vi "configure dialog.vi"(9 "Channel":u32, 11 "Attributes in":T1[](array[typedef])) -> (1 "Channel out":u32, 2 "Cancelled?":bool, 3 "Attributes out":T1[](array[typedef]))   [LabVIEW 2020, in "Set DDT Attributes.lvlib"]
doc: "Sets the attributes of the dynamic data you wire to <B>Signals In</B>."
uses:
  <vilib>/express/express signal manip/GetorSetDDTAttributes/Set DDT Attributes/Set DDT Attributes.lvlib
  <vilib>/express/express signal manip/GetorSetDDTAttributes/Shared VIs/Attributes data.ctl
  <vilib>/express/express signal manip/GetorSetDDTAttributes/Shared VIs/Input.ctl
  <vilib>/express/express signal manip/GetorSetDDTAttributes/Shared VIs/Attributes name.ctl
  <vilib>/express/express signal manip/GetorSetDDTAttributes/Shared VIs/TimeType.ctl
  <vilib>/express/express signal manip/GetorSetDDTAttributes/Shared VIs/XDimension.ctl
  <vilib>/express/express signal manip/GetorSetDDTAttributes/Shared VIs/GetSetShared.lvlib
  <vilib>/express/express signal manip/GetorSetDDTAttributes/Set DDT Attributes/Set DDT Properties.xnode
panel:
  in  "Signal Index":u32
  in  "Start timestamp":bool
  in  "Unit":bool
  in  "X dimension":bool
  in  "Timestamp":bool
  in  "Time mode":bool
  in  "Signal name":bool
  in  "Timestamp value":timestamp
  in  "Start timestamp value":timestamp
  in  "Unit value":string
  in  "Time mode value":u16(ring)=1 items=["Absolute", "Relative"]
  in  "X dimension value":u16(ring)=1 items=["No Unit [-]", "Time [sec]", "Frequency [Hz]"]
  in  "Signal name value":string
  in  "help":bool
  in  "Cancel":bool
  in  "OK":bool
  # "All Signals"
  # "Value"
  # "Value"
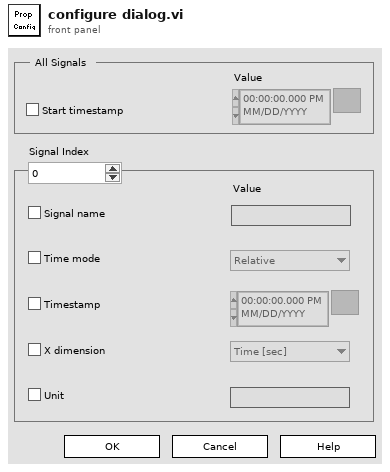
[diagram p1: front panel]
types:
  T1 = typedef "GetSetShared.lvlib/Attributes data.ctl" = cluster{"State":T2, "Attributes Name":T3, "Value":variant, "wired?":bool}
  T2 = typedef "GetSetShared.lvlib/Input.ctl" = bool
  T3 = typedef "GetSetShared.lvlib/Attributes name.ctl" = enum16{"NI_ChannelName", "NI_ExpIsRelativeTime", "NI_ExpTimeStamp", "NI_ExpStartTimeStamp", "NI_ExpXDimension", "NI_UnitDescription"}
  T4 = typedef "GetSetShared.lvlib/TimeType.ctl" = enum16{"Absolute", "Relative"}
  T5 = typedef "GetSetShared.lvlib/XDimension.ctl" = enum16{"No Unit [-]", "Time [sec]", "Frequency [Hz]"}
  T6 = cluster{"Description":string, "Path":path, "Tag":string}
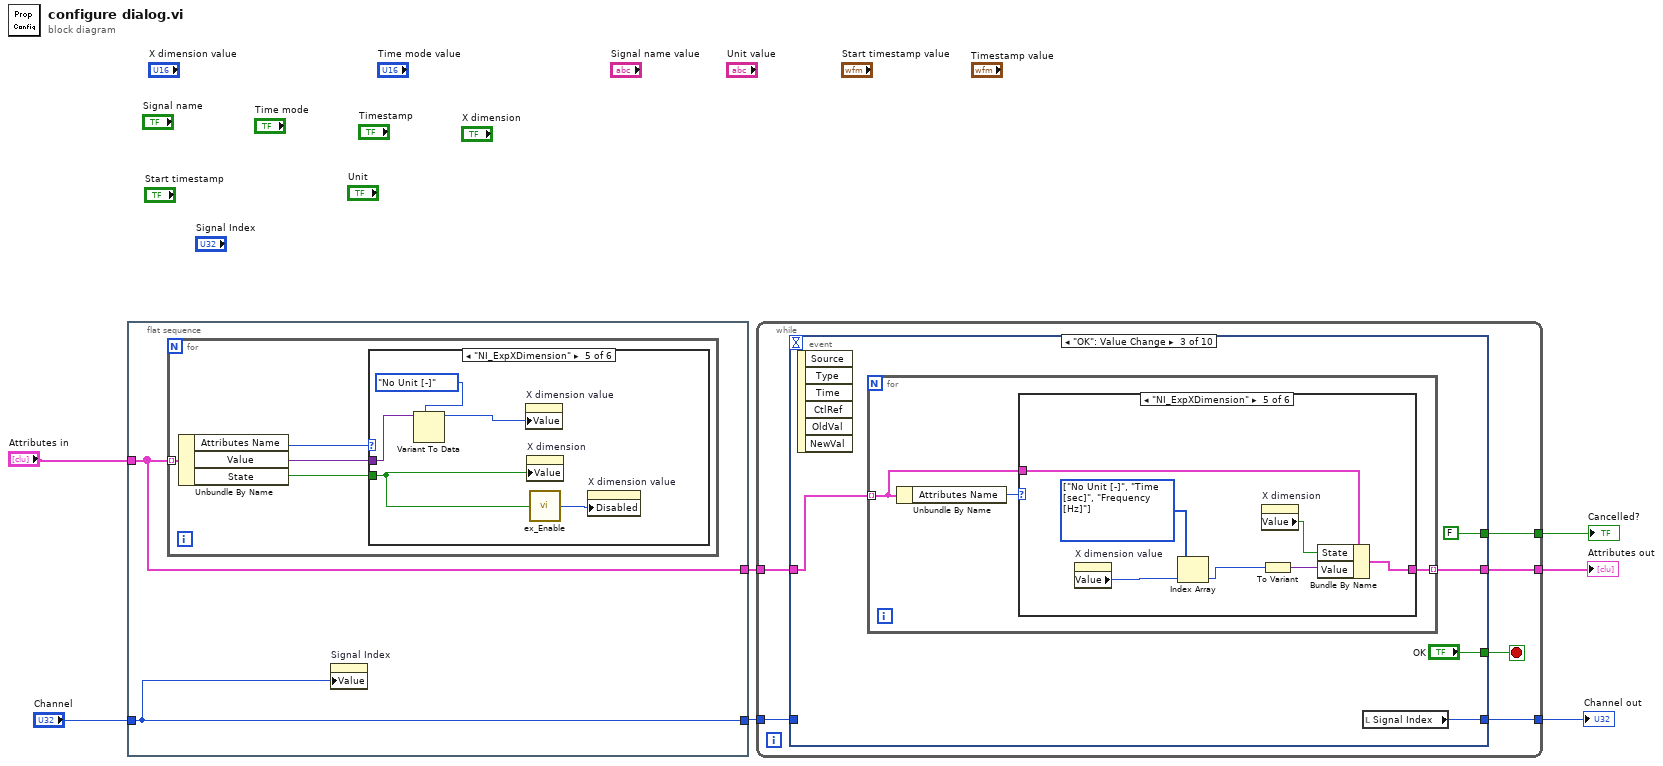
[diagram p0: block diagram]
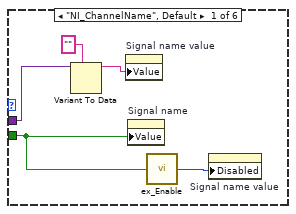
[diagram p2: hidden frame]
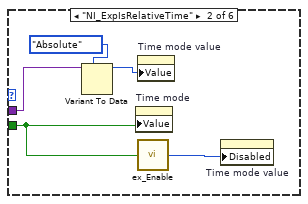
[diagram p3: hidden frame]
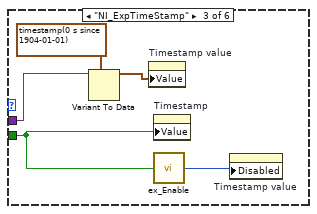
[diagram p4: hidden frame]
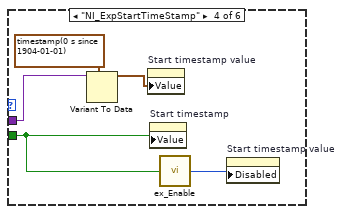
[diagram p5: hidden frame]
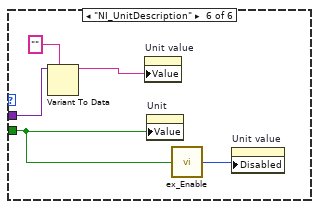
[diagram p6: hidden frame]
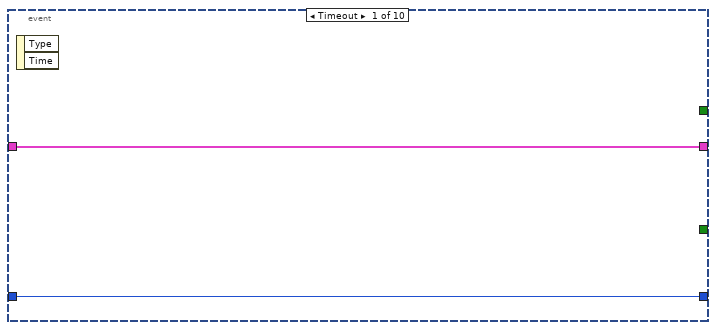
[diagram p7: hidden frame]
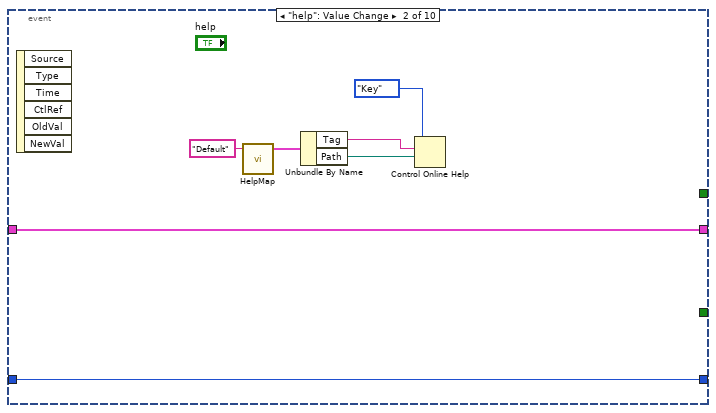
[diagram p8: hidden frame]
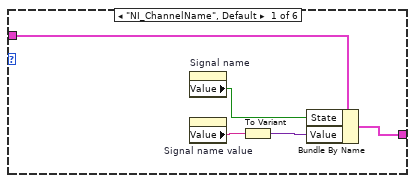
[diagram p9: hidden frame]
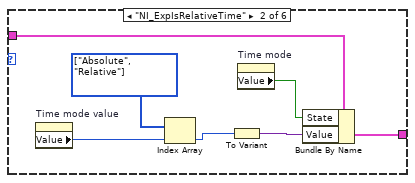
[diagram p10: hidden frame]
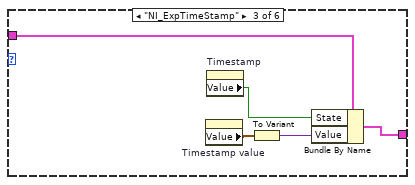
[diagram p11: hidden frame]
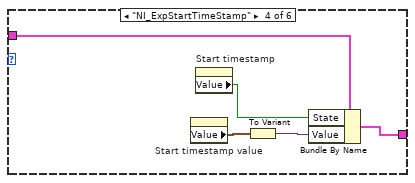
[diagram p12: hidden frame]
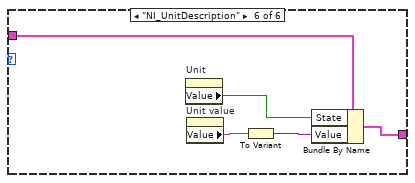
[diagram p13: hidden frame]
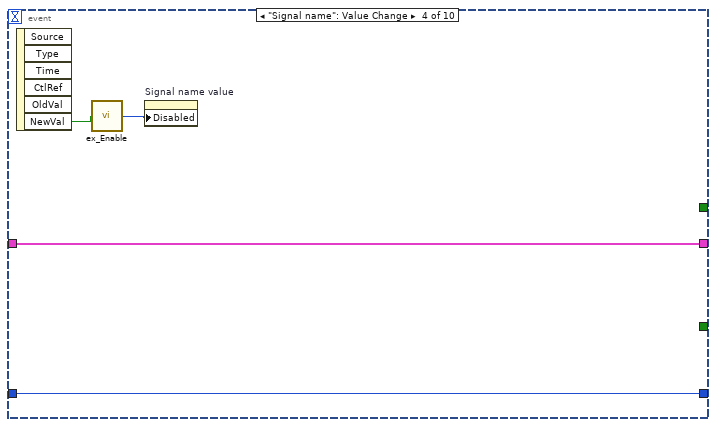
[diagram p14: hidden frame]
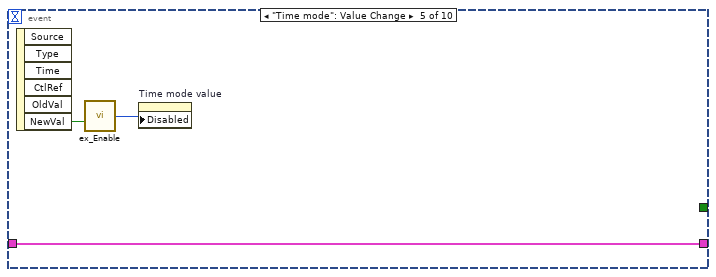
[diagram p15: hidden frame]
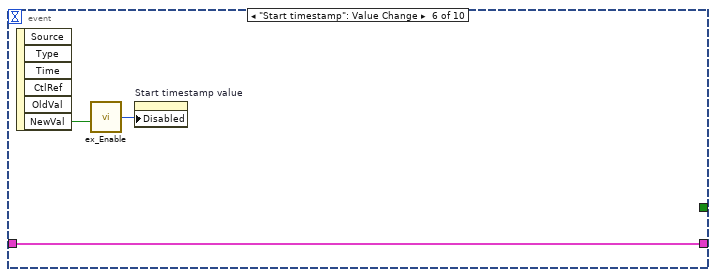
[diagram p16: hidden frame]
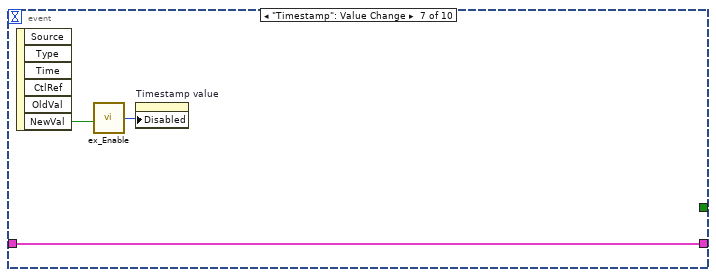
[diagram p17: hidden frame]
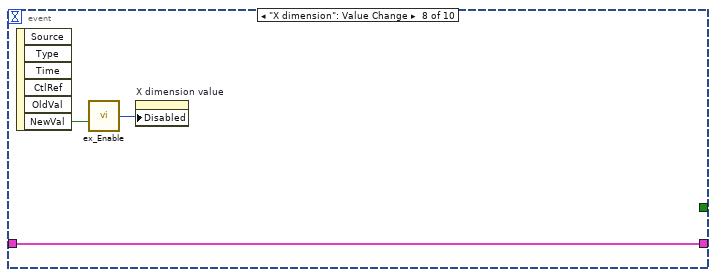
[diagram p18: hidden frame]
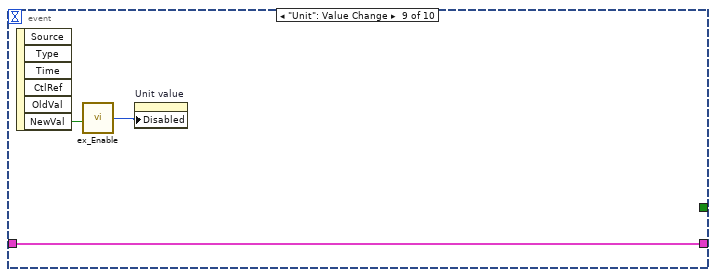
[diagram p19: hidden frame]
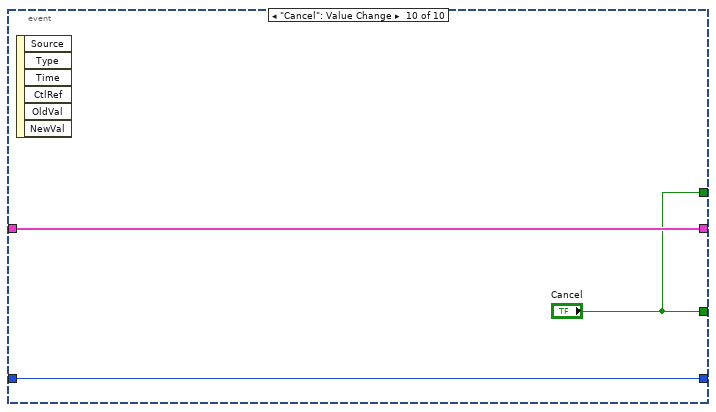
[diagram p20: hidden frame]
diagram:
  n1 = flat-sequence {
    tunnel: "Attributes in" -> [w9]
    tunnel: [w9] -> w4
    tunnel: "Channel" -> [w8]
    tunnel: [w8] -> w3
    frame #0 {
      n2 = for {
        tunnel: w9 -> [w13] mode=indexing
        n3 = Unbundle By Name(w13) -> ("Attributes Name"=w12:T3, "Value"=w11:variant, "State"=w10:T2)
        n4 = case shown="\"NI_ExpXDimension\"" w12 {
          tunnel: w11 -> [w18 w23 w28 w32 w38 w43]
          tunnel: w10 -> [w14 w21 w24 w29 w34 w39]
          frame "NI_ChannelName", Default {
            n5 = Variant To Data(type="", Variant=w18) -> (data=w16:string)  [unwired: 1 in, 1 out]
            n6 = property on="Signal name value" class="Str"("Value"=w16) -> ()  [unwired: 2 in, 2 out]
            n7 = property on="Signal name" class="Bool (strict)"("Value"=w14) -> ()  [unwired: 2 in, 2 out]
            n8 = call <vilib>:"ex_Enable.vi"("Enable?"=w14) -> ("Disabled Value"=w15:u8)
            n9 = property on="Signal name value" class="Str"("Disabled"=w15) -> ()  [unwired: 2 in, 2 out]
          }
          frame "NI_ExpIsRelativeTime" {
            n10 = Variant To Data(type=TimeType."Absolute" ("RelativeTime?"), Variant=w23) -> (data=w19:T4)  [unwired: 1 in, 1 out]
            n11 = property on="Time mode" class="Bool (strict)"("Value"=w21) -> ()  [unwired: 2 in, 2 out]
            n12 = property on="Time mode value" class="Ring (strict)"("Value"=w19) -> ()  [unwired: 2 in, 2 out]
            n13 = call <vilib>:"ex_Enable.vi"("Enable?"=w21) -> ("Disabled Value"=w22:u8)
            n14 = property on="Time mode value" class="Ring (strict)"("Disabled"=w22) -> ()  [unwired: 2 in, 2 out]
          }
          frame "NI_ExpTimeStamp" {
            n15 = Variant To Data(type=timestamp(0 s since 1904-01-01), Variant=w28) -> (data=w26:timestamp)  [unwired: 1 in, 1 out]
            n16 = property on="Timestamp value" class="AbsTime (strict)"("Value"=w26) -> ()  [unwired: 2 in, 2 out]
            n17 = property on="Timestamp" class="Bool (strict)"("Value"=w24) -> ()  [unwired: 2 in, 2 out]
            n18 = call <vilib>:"ex_Enable.vi"("Enable?"=w24) -> ("Disabled Value"=w25:u8)
            n19 = property on="Timestamp value" class="AbsTime (strict)"("Disabled"=w25) -> ()  [unwired: 2 in, 2 out]
          }
          frame "NI_ExpStartTimeStamp" {
            n20 = Variant To Data(type=timestamp(0 s since 1904-01-01), Variant=w32) -> (data=w31:timestamp)  [unwired: 1 in, 1 out]
            n21 = property on="Start timestamp value" class="AbsTime (strict)"("Value"=w31) -> ()  [unwired: 2 in, 2 out]
            n22 = property on="Start timestamp" class="Bool (strict)"("Value"=w29) -> ()  [unwired: 2 in, 2 out]
            n23 = call <vilib>:"ex_Enable.vi"("Enable?"=w29) -> ("Disabled Value"=w30:u8)
            n24 = property on="Start timestamp value" class="AbsTime (strict)"("Disabled"=w30) -> ()  [unwired: 2 in, 2 out]
          }
          frame "NI_ExpXDimension" {
            n25 = Variant To Data(type=XDimension."No Unit [-]" ("XDimension"), Variant=w38) -> (data=w35:T5)  [unwired: 1 in, 1 out]
            n26 = property on="X dimension value" class="Ring (strict)"("Value"=w35) -> ()  [unwired: 2 in, 2 out]
            n27 = property on="X dimension" class="Bool (strict)"("Value"=w34) -> ()  [unwired: 2 in, 2 out]
            n28 = call <vilib>:"ex_Enable.vi"("Enable?"=w34) -> ("Disabled Value"=w37:u8)
            n29 = property on="X dimension value" class="Ring (strict)"("Disabled"=w37) -> ()  [unwired: 2 in, 2 out]
          }
          frame "NI_UnitDescription" {
            n30 = Variant To Data(type="", Variant=w43) -> (data=w41:string)  [unwired: 1 in, 1 out]
            n31 = property on="Unit value" class="Str"("Value"=w41) -> ()  [unwired: 2 in, 2 out]
            n32 = property on="Unit" class="Bool (strict)"("Value"=w39) -> ()  [unwired: 2 in, 2 out]
            n33 = call <vilib>:"ex_Enable.vi"("Enable?"=w39) -> ("Disabled Value"=w40:u8)
            n34 = property on="Unit value" class="Str"("Disabled"=w40) -> ()  [unwired: 2 in, 2 out]
          }
        }
      }
      n35 = property on="Signal Index" class="DigNum (strict)"("Value"=w8) -> ()  [unwired: 2 in, 2 out]
    }
  }
  n36 = while {
    tunnel: [w48] -> w7
    tunnel: w4 -> [w47]
    tunnel: [w46] -> w6
    tunnel: w3 -> [w44]
    tunnel: [w45] -> w5
    stop <- w49 stop-if-true
    n37 = event shown="[2] \"OK\": Value Change" {
      selector: _ -> [_ _ _ _ _ _ _ _ _ _]
      dyn-events: _ -> [_ _ _ _ _ _ _ _ _ _]
      timeout: _ -> [_ _ _ _ _ _ _ _ _ _]
      tunnel: [_ _ "OK" _ _ _ _ _ _ "Cancel"] -> w49
      tunnel: [_ _ FALSE ("Cancel") _ _ _ _ _ _ "Cancel"] -> w48
      tunnel: w47 -> [w50 w57 w62 w103 w105 w108 w111 w114 w117 w121]
      tunnel: [w50 w57 w61 w103 w105 w108 w111 w114 w117 w121] -> w46
      tunnel: [w51 w58 w60 w104 _ _ _ _ _ w122] -> w45
      tunnel: w44 -> [w51 w58 _ w104 _ _ _ _ _ w122]
      event Timeout {
        n38 = event-data() -> ()  [unwired: 3 out]
      }
      event "help": Value Change {
        n39 = event-data() -> ()  [unwired: 7 out]
        n40 = call <vilib>:"HelpMap.vi"("Standard Help ID"="Default") -> ("Standard Help Info"=w54:T6)  [unwired: 2 in, 2 out]
        n41 = Unbundle By Name(w54) -> ("Tag"=w53:string, "Path"=w52:path)
        n42 = Control Online Help(2:w52, 3:w53, 4:enum16{"Contents", "Key", "Close"}."Key" ("Operation")) -> ()  [unwired: 1 in, 1 out]
      }
      event "OK": Value Change {
        n43 = event-data() -> ()  [unwired: 7 out]
        n44 = for {
          tunnel: w62 -> [w66] mode=indexing
          tunnel: [w65] -> w61 mode=indexing
          n45 = Unbundle By Name(w66) -> ("Attributes Name"=w64:T3)
          n46 = case shown="\"NI_ExpXDimension\"" w64 {
            tunnel: w66 -> [w68 w76 w80 w85 w93 w97]
            tunnel: [w70 w78 w82 w87 w95 w100] -> w65
            frame "NI_ChannelName", Default {
              n47 = property on="Signal name" class="Bool (strict)"() -> ("Value"=w67:bool)  [unwired: 2 in, 2 out]
              n48 = property on="Signal name value" class="Str"() -> ("Value"=w69:string)  [unwired: 2 in, 2 out]
              n49 = To Variant(anything=w69) -> (Variant=w71:variant)
              n50 = Bundle By Name(cluster=w68, "State"=w67, "Value"=w71) -> (w70:T1)
            }
            frame "NI_ExpIsRelativeTime" {
              w74 = T4[] [enum."Absolute", enum."Relative"] items=["Absolute", "Relative"] ("Array")
              n51 = property on="Time mode value" class="Ring (strict)"() -> ("Value"=w73:u16)  [unwired: 2 in, 2 out]
              n52 = Index Array(array=w74, index=w73) -> (element=w72:T4)
              n53 = To Variant(anything=w72) -> (Variant=w77:variant)
              n54 = property on="Time mode" class="Bool (strict)"() -> ("Value"=w75:bool)  [unwired: 2 in, 2 out]
              n55 = Bundle By Name(cluster=w76, "State"=w75, "Value"=w77) -> (w78:T1)
            }
            frame "NI_ExpTimeStamp" {
              n56 = property on="Timestamp value" class="AbsTime (strict)"() -> ("Value"=w81:timestamp)  [unwired: 2 in, 2 out]
              n57 = property on="Timestamp" class="Bool (strict)"() -> ("Value"=w79:bool)  [unwired: 2 in, 2 out]
              n58 = To Variant(anything=w81) -> (Variant=w83:variant)
              n59 = Bundle By Name(cluster=w80, "State"=w79, "Value"=w83) -> (w82:T1)
            }
            frame "NI_ExpStartTimeStamp" {
              n60 = property on="Start timestamp value" class="AbsTime (strict)"() -> ("Value"=w86:timestamp)  [unwired: 2 in, 2 out]
              n61 = property on="Start timestamp" class="Bool (strict)"() -> ("Value"=w84:bool)  [unwired: 2 in, 2 out]
              n62 = To Variant(anything=w86) -> (Variant=w88:variant)
              n63 = Bundle By Name(cluster=w85, "State"=w84, "Value"=w88) -> (w87:T1)
            }
            frame "NI_ExpXDimension" {
              w91 = T5[] [enum."No Unit [-]", enum."Time [sec]", enum."Frequency [Hz]"] items=["No Unit [-]", "Time [sec]", "Frequency [Hz]"] ("Array")
              n64 = property on="X dimension value" class="Ring (strict)"() -> ("Value"=w90:u16)  [unwired: 2 in, 2 out]
              n65 = Index Array(array=w91, index=w90) -> (element=w89:T5)
              n66 = property on="X dimension" class="Bool (strict)"() -> ("Value"=w92:bool)  [unwired: 2 in, 2 out]
              n67 = To Variant(anything=w89) -> (Variant=w94:variant)
              n68 = Bundle By Name(cluster=w93, "State"=w92, "Value"=w94) -> (w95:T1)
            }
            frame "NI_UnitDescription" {
              n69 = property on="Unit" class="Bool (strict)"() -> ("Value"=w96:bool)  [unwired: 2 in, 2 out]
              n70 = property on="Unit value" class="Str"() -> ("Value"=w98:string)  [unwired: 2 in, 2 out]
              n71 = To Variant(anything=w98) -> (Variant=w99:variant)
              n72 = Bundle By Name(cluster=w97, "State"=w96, "Value"=w99) -> (w100:T1)
            }
          }
        }
        n73 = local read "Signal Index"() -> (w60:u32)
      }
      event "Signal name": Value Change {
        n74 = event-data() -> ("NewVal"=w102:bool)  [unwired: 6 out]
        n75 = call <vilib>:"ex_Enable.vi"("Enable?"=w102) -> ("Disabled Value"=w101:u8)
        n76 = property on="Signal name value" class="Str"("Disabled"=w101) -> ()  [unwired: 2 in, 2 out]
      }
      event "Time mode": Value Change {
        n77 = event-data() -> ("NewVal"=w107:bool)  [unwired: 6 out]
        n78 = call <vilib>:"ex_Enable.vi"("Enable?"=w107) -> ("Disabled Value"=w106:u8)
        n79 = property on="Time mode value" class="Ring (strict)"("Disabled"=w106) -> ()  [unwired: 2 in, 2 out]
      }
      event "Start timestamp": Value Change {
        n80 = event-data() -> ("NewVal"=w110:bool)  [unwired: 6 out]
        n81 = call <vilib>:"ex_Enable.vi"("Enable?"=w110) -> ("Disabled Value"=w109:u8)
        n82 = property on="Start timestamp value" class="AbsTime (strict)"("Disabled"=w109) -> ()  [unwired: 2 in, 2 out]
      }
      event "Timestamp": Value Change {
        n83 = event-data() -> ("NewVal"=w113:bool)  [unwired: 6 out]
        n84 = call <vilib>:"ex_Enable.vi"("Enable?"=w113) -> ("Disabled Value"=w112:u8)
        n85 = property on="Timestamp value" class="AbsTime (strict)"("Disabled"=w112) -> ()  [unwired: 2 in, 2 out]
      }
      event "X dimension": Value Change {
        n86 = event-data() -> ("NewVal"=w116:bool)  [unwired: 6 out]
        n87 = call <vilib>:"ex_Enable.vi"("Enable?"=w116) -> ("Disabled Value"=w115:u8)
        n88 = property on="X dimension value" class="Ring (strict)"("Disabled"=w115) -> ()  [unwired: 2 in, 2 out]
      }
      event "Unit": Value Change {
        n89 = event-data() -> ("NewVal"=w119:bool)  [unwired: 6 out]
        n90 = call <vilib>:"ex_Enable.vi"("Enable?"=w119) -> ("Disabled Value"=w118:u8)
        n91 = property on="Unit value" class="Str"("Disabled"=w118) -> ()  [unwired: 2 in, 2 out]
      }
      event "Cancel": Value Change {
        n92 = event-data() -> ()  [unwired: 7 out]
      }
    }
  }
  "Cancelled?" <- w7
  "Attributes out" <- w6
  "Channel out" <- w5
